vi "Zero_One_Loss.vi"(6 "Type y_pred":T1(ring), 7 "Type y_true":T1(ring), 8 "error in (no error)":errorcluster caption="entrée d'erreur (pas d'erreur)", 9 "y_pred":string[][](array[string]), 10 "y_true":string[][](array[string]), 11 "zero_one_loss":cluster{"normalize":bool, "sample_weight":dbl[]}={"normalize"=TRUE, "sample_weight"=[]}) -> (0 "error out":errorcluster caption="sortie d'erreur", 3 "Score":string)   [LabVIEW 2020]
doc: "Zero-one classification loss.\n\nIf normalize is True, return the fraction of misclassifications (float), else it returns the number of misclassifications (int). The best performance is 0.\n\n\n\nParameters : \n\n- y_true : 1d array-like, or label indicator array / sparse matrix\nGround truth (correct) labels.\n\n- y_pred : 1d array-like, or label indicator array / sparse matrix\nPredicted labels, as returned by a classifier.\n\n- normalize : bool, optional (default=True)\nIf False, return the number of misclassifications. Otherwise, return the fraction of misclassifications.\n\n- sample_weight : array-like of shape (n_samples,), default=None\nSample weights.\n\nReturns : \n\n- loss : float or int,\nIf normalize == True, return the fraction of misclassifications (float), else it returns the number of misclassifications (int)."
uses:
  Zero_One_Loss.lvclass
panel:
  out "Zero_One_Loss.lvclass":refnum<class "Zero_One_Loss.lvclass">
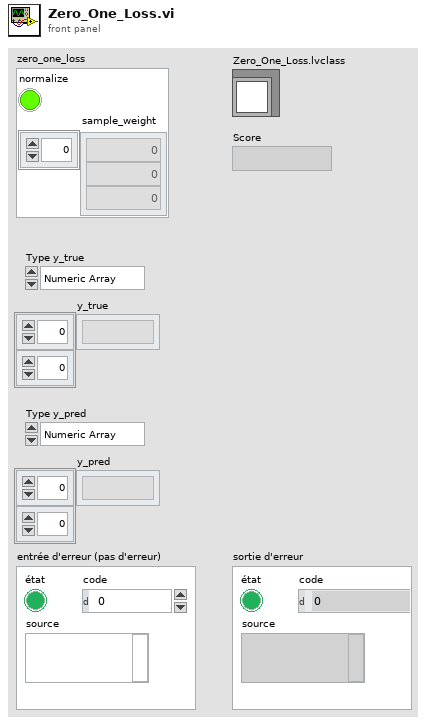
[diagram p1: front panel]
types:
  T1 = enum16{"Numeric Array", "String Array", "Sparse"}
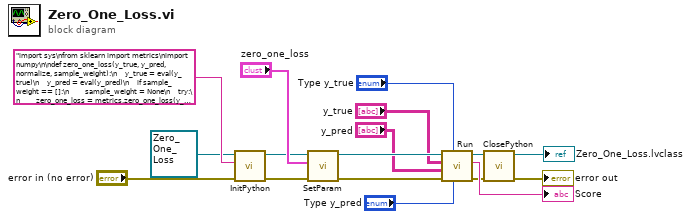
[diagram p0: block diagram]
diagram:
  n1 = call-dynamic "InitPython.vi"("error in (no error)"="error in (no error)", "Python Instruction"="import sys\nfrom sklearn import metrics\nimport numpy\n\ndef zero_one_loss(y_true, y_pred, normalize, sample_weight):\n    y_true = eval(y_true)\n    y_pred = eval(y_pred)\n    if sample_weight == []:\n        sample_weight = None\n    try:\n        zero_one_loss = metrics.zero_one_loss(y_true, y_pred, normalize, sample_weight)\n        zero_one_loss = zero_one_loss.tolist()\n        return str(zero_one_loss)\n    except:\n        erreur = sys.exc_info()\n        typerr = u\"%s\" % (erreur[0])\n        typerr = typerr[typerr.find(\"'\")+1:typerr.rfind(\"'\")]\n        msgerr = u\"%s\" % (erreur[1])\n        message = str('/!\\\\ {0} : {1}'. format(typerr,msgerr))\n        return message", "Scikit-learn en entrée"=refnum<class "Zero_One_Loss.lvclass"> refnum ("Zero_One_Loss.lvclass")) -> ("error out"=w13:errorcluster, "Scikit-learn en sortie"=w11:refnum<class "Zero_One_Loss.lvclass">)  [unwired: 7 in]
  n2 = call-dynamic "SetParam.vi"("error in (no error)"=w13, "zero_one_loss"="zero_one_loss", "Zero_One_Loss.lvclass"=w11) -> ("error out"=w7:errorcluster, "Zero_One_Loss.lvclass"=w10:refnum<class "Zero_One_Loss.lvclass">)  [unwired: 7 in]
  n3 = call-dynamic "Run.vi"("Type y_pred"="Type y_pred", "Type y_true"="Type y_true", "error in (no error)"=w7, "y_pred"="y_pred", "y_true"="y_true", "Zero_One_Loss.lvclass"=w10) -> ("error out"=w5:errorcluster, "String Data"=→"Score":string, "Zero_One_Loss.lvclass"=w9:refnum<class "Zero_One_Loss.lvclass">)  [unwired: 3 in]
  n4 = call-dynamic "ClosePython.vi"("error in (no error)"=w5, "Scikit-learn en entrée"=w9) -> ("error out"=→"error out":errorcluster, "Scikit-learn en sortie"=→"Zero_One_Loss.lvclass":refnum<class "Zero_One_Loss.lvclass">)  [unwired: 8 in]
